vi "MakeCameraDataString.vi"(1 "Image StDev":dbl format="%.6f", 2 "DC Offset":dbl format="%.6f", 3 "Saved Frame Number":dbl format="%.6f", 4 "Frame Number":dbl format="%.6f") -> (0 "Output String":string)   [LabVIEW 2013]
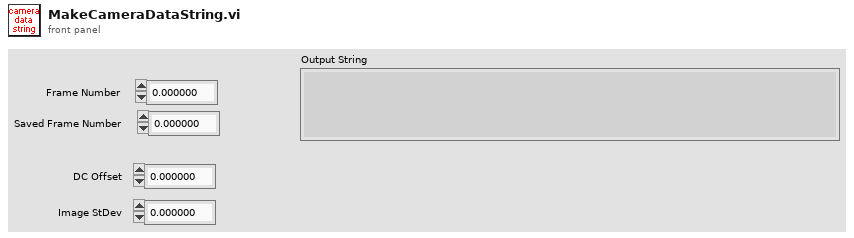
[diagram p1: front panel]
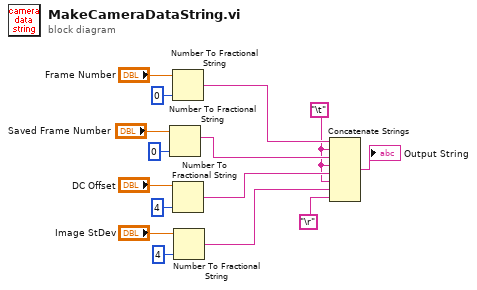
[diagram p0: block diagram]
diagram:
  w1 = "\t"
  n1 = Number To Fractional String(number="Saved Frame Number", precision (6)=i16 0) -> (F-format string=w2:string)  [unwired: 2 in]
  n2 = Number To Fractional String(number="Frame Number", precision (6)=i16 0) -> (F-format string=w3:string)  [unwired: 2 in]
  n3 = Number To Fractional String(number="DC Offset", precision (6)=i16 4) -> (F-format string=w8:string)  [unwired: 2 in]
  n4 = Number To Fractional String(number="Image StDev", precision (6)=i16 4) -> (F-format string=w7:string)  [unwired: 2 in]
  n5 = Concatenate Strings(w3, w1, w2, w1, w8, w1, w7, "\r") -> (→"Output String":string)
